vi "Result.vi"(8 "error in (no error)":errorcluster, 10 "Result":T1={"Name"="", "Description"="", "Status"=enum."Passed", "Result Type"=enum."Test Suite", "Execution Time"=0.0, "Data"={"Expected"=variant, "Actual"=variant, "Delta"=variant}}, 11 "Report Generator In":refnum<class "Report Generator.lvclass">) -> (0 "error out":errorcluster)   [LabVIEW 2020, in "Reports.lvlib" / "Report Generator.lvclass"]
uses:
  Report Generator.lvclass
  C:/git/astemes-lunit/source/User Interface/Process/Process.lvclass
  Core/Result/Result.ctl
  Core/Result/Status.ctl
  Core/Result/Type.ctl
  User Interface/Process/Process.lvclass/Process.ctl
  User Interface/Process/Process.lvclass
  Core/Result/Result.lvlib
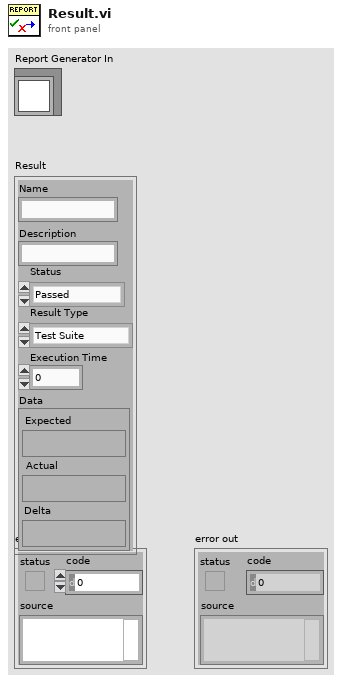
[diagram p1: front panel]
types:
  T1 = typedef "Result.lvlib/Result.ctl" = cluster{"Name":string, "Description":string, "Status":T2, "Result Type":T3, "Execution Time":dbl, "Data":cluster{"Expected":variant, "Actual":variant, "Delta":variant}}
  T2 = typedef "Result.lvlib/Status.ctl" = enum16{"", "Passed", "Failed", "Error", "Skipped", "Setup Error", "Broken", "Teardown Error"}
  T3 = typedef "Result.lvlib/Type.ctl" = enum16{"Test Case", "Test Suite", "Test Run", "Pass", "Fail", "Skip", "Pass if", "Fail if", "Pass if Error", "Fail if Error", "Pass if Equal", "Fail if Equal"}
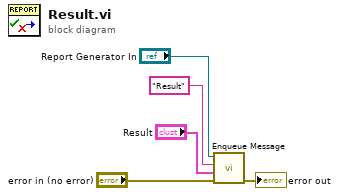
[diagram p0: block diagram]
diagram:
  n1 = call "Enqueue Message.vi"("error in (no error)"="error in (no error)", "Message Data"="Result", "Message"="Result", "Process In"="Report Generator In") -> ("error out"=→"error out":errorcluster)  [unwired: 6 in, 1 out]
